vi "Manual Assembly_2.vi"() -> ()   [LabVIEW 2016]
uses:
  Classes/Routine/Routine Enum.ctl
  Classes/Routine/Settings.ctl
  Classes/Assembly/Assembly Run.lvclass
  Classes/Workspace/Fixture Enum.ctl
  Classes/Controller/Controller.lvclass
  Classes/Workspace/Fixture.lvclass
  Classes/Routine/Routine.lvclass
panel:
  in  "Routine type":T1(ring)
  in  "inistialize BT":bool
  out "inistialize":bool
  in  "Routine n":T2(ring)
  in  "Settings":T3
  in  "?":bool
  in  "Update":bool
  in  "Stage":i32(listbox)=-1
  in  "Routine":T4=enum."Dispense on Plate"
  in  "Stop":bool
  in  "Remove":bool
  in  "Add":bool
  in  "Go":bool
  # "6 Inch"
  # "8 Inch"
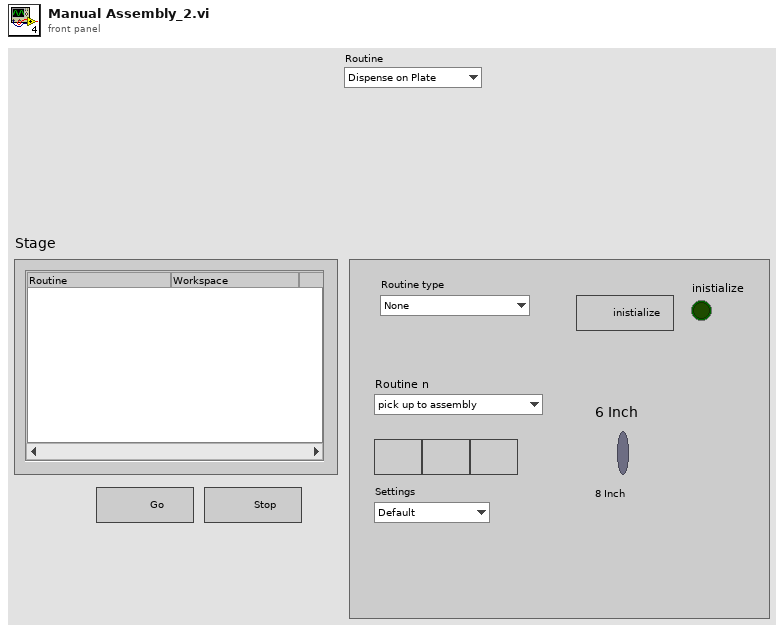
[diagram p1: front panel]
types:
  T1 = enum16{"None", "Kapton assembly", "sensor assembly", "PCB assembly2", "PCB assembly", "Pick up and Put down", "baseplate dispense", "sensor dispense", "sensor dispense2"}
  T2 = enum16{"pick up to assembly", "put down pick up tool", "Primary Pick Up", "Pick Up All", "Put Down Secondary", "Put Down All", "Release Syringe", "Secondary Pick Up", "Secure Syringe", "Dispense on Plate", "Dispense on Kapton", "Dispense on Sensor", "Dispense on Sensor2"}
  T3 = typedef "Routine.lvclass/Settings.ctl" = enum16{"Default", "Custom"}
  T4 = typedef "Routine.lvclass/Routine Enum.ctl" = enum16{"Primary Pick Up", "Pick Up All", "Put Down Secondary", "Put Down All", "Release Syringe", "Secondary Pick Up", "Secure Syringe", "Dispense on Plate", "Dispense on Kapton", "Dispense on Sensor", "Dispense on Sensor2"}
  T5 = typedef "Fixture.lvclass/Fixture Enum.ctl" = enum16{"Assembly Tray", "Syringe Space", "Component", "Pick Up Tool", "Current Position"}
  T6 = enum16{"pick up to assembly", "put down pick up tool", "Primary Pick Up", "Pick Up All", "Put Down Secondary", "Put Down All", "Release Syringe", "Secondary Pick Up", "Secure Syringe", "Dispense on Plate", "Dispense on Kapton", "Dispense on Sensor", "Dispense on Sensor2"}[]
  T7 = typedef "Controller.lvclass/Controllers.ctl" = cluster{"I-O.lvclass":refnum<class "I-O.lvclass">, "Motion.lvclass":refnum<class "Motion.lvclass">, "Dispenser.lvclass":refnum<class "Dispenser.lvclass">}
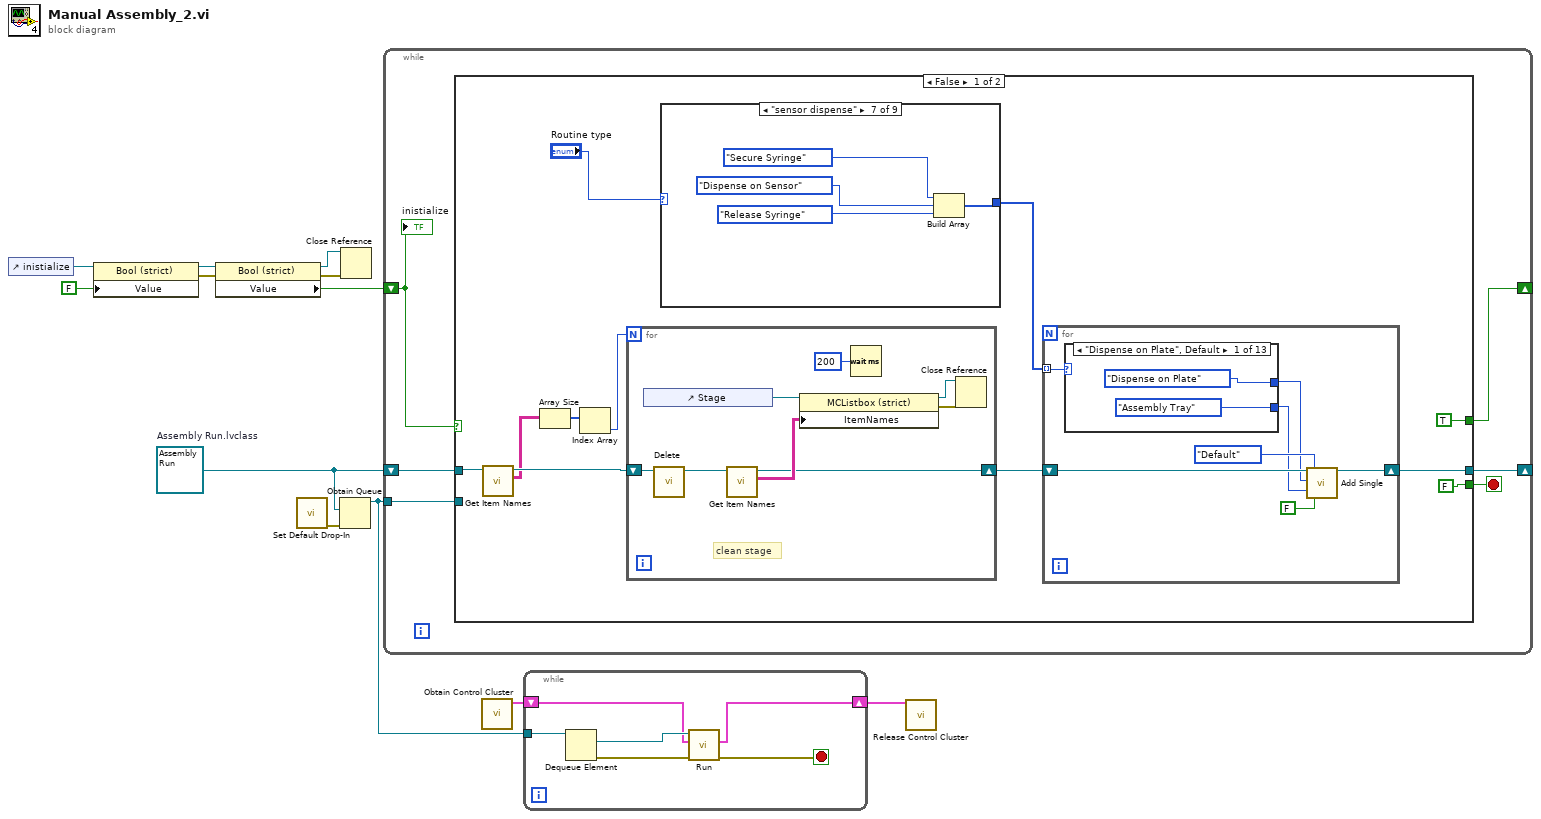
[diagram p0: block diagram]
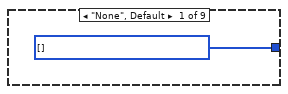
[diagram p2: hidden frame]
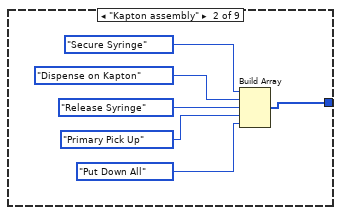
[diagram p3: hidden frame]
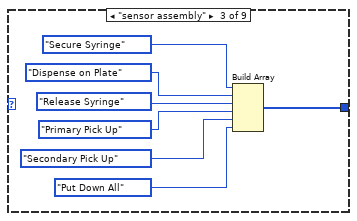
[diagram p4: hidden frame]
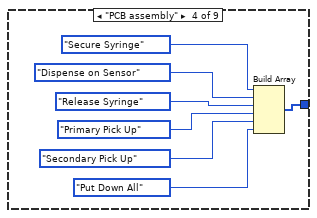
[diagram p5: hidden frame]
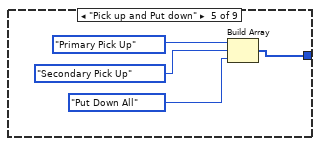
[diagram p6: hidden frame]
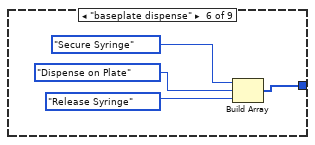
[diagram p7: hidden frame]
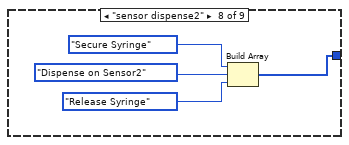
[diagram p8: hidden frame]
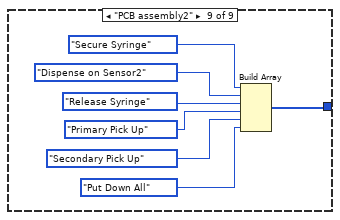
[diagram p9: hidden frame]
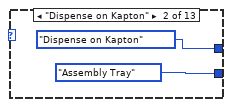
[diagram p10: hidden frame]
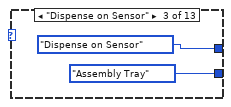
[diagram p11: hidden frame]
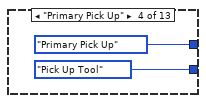
[diagram p12: hidden frame]
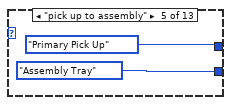
[diagram p13: hidden frame]
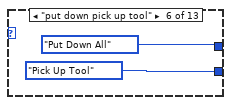
[diagram p14: hidden frame]
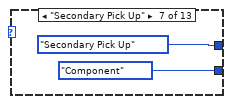
[diagram p15: hidden frame]
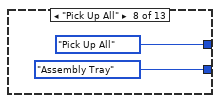
[diagram p16: hidden frame]
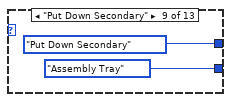
[diagram p17: hidden frame]
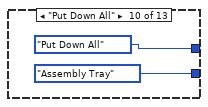
[diagram p18: hidden frame]
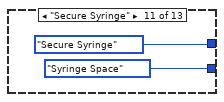
[diagram p19: hidden frame]
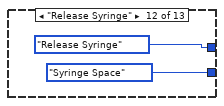
[diagram p20: hidden frame]
diagram:
  w8 = refnum<class "Assembly Run.lvclass"> refnum  # Assembly Run.lvclass
  n1 = control-ref of="inistialize"() -> (w2:refnum<vi>)
  n2 = property class="Bool (strict)"(reference=w2, "Value"=FALSE) -> (reference out=w4:refnum<vi>, error out=w3:errorcluster)  [unwired: 1 in]
  n3 = property class="Bool (strict)"(reference=w4, error in=w3) -> (reference out=w5:refnum<vi>, error out=w6:errorcluster, "Value"=w7:bool)
  n4 = call "Set Default Drop-In.vi"() -> ("error out"=w9:errorcluster)  [unwired: 11 in]
  n5 = Obtain Queue(element data type=w8, error in (no error)=w9) -> (queue out=w12:refnum<queue>)  [unwired: 3 in, 2 out]
  n6 = Close Reference(reference=w5, error in (no error)=w6) -> ()  [unwired: 1 out]
  n7 = while {
    shift-right: [w15] -> _
    shift-left: w8 -> [w16]
    tunnel: w12 -> [w17]
    shift-right: [w13] -> _
    shift-left: w7 -> [w14]
    stop <- w18 stop-if-true
    n8 = case shown="False" w14 {
      selector: w14 -> [_ w117]
      tunnel: [FALSE w125] -> w18
      tunnel: w17 -> [_ w124]
      tunnel: w16 -> [w26 w121]
      tunnel: [w21 w119] -> w15
      tunnel: [TRUE w118] -> w13
      frame False {
        n9 = call "Get Item Names.vi"("Assembly Run in"=w26) -> ("Item names"=w25:string[][], "Assembly Run out"=w27:refnum<class "Assembly Run.lvclass">)  [unwired: 8 in, 1 out]
        n10 = Array Size(array=w25) -> (size(s)=w24:i32[])
        n11 = Index Array(array=w24) -> (element=w23:i32)  [unwired: 1 in]
        n12 = for {
          N: w23 -> [_]
          shift-right: [w108] -> w22
          shift-left: w27 -> [w110]
          # "clean stage"
          n13 = control-ref of="Stage"() -> (w107:refnum<vi>)
          n14 = call "Delete.vi"("Assembly In"=w110) -> ("Assembly Out"=w109:refnum<class "Assembly Run.lvclass">)  [unwired: 9 in, 1 out]
          n15 = call "Get Item Names.vi"("Assembly Run in"=w109) -> ("Item names"=w113:string[][], "Assembly Run out"=w108:refnum<class "Assembly Run.lvclass">)  [unwired: 8 in, 1 out]
          n16 = property class="MCListbox (strict)"(reference=w107, "ItemNames"=w113) -> (reference out=w114:refnum<vi>, error out=w112:errorcluster)  [unwired: 1 in]
          n17 = Wait (ms)(milliseconds to wait=u32 200) -> ()  [unwired: 1 out]
          n18 = Close Reference(reference=w114, error in (no error)=w112) -> ()  [unwired: 1 out]
        }
        n19 = case shown="\"sensor dispense\"" "Routine type" {
          tunnel: [w30 w36 w43 w50 w54 w58 w62 w66 w73] -> w19
          frame "None", Default {
            w30 = T6 [] items=["pick up to assembly", "put down pick up tool", "Primary Pick Up", "Pick Up All", "Put Down Secondary", "Put Down All", "Release Syringe", "Secondary Pick Up", "Secure Syringe", "Dispense on Plate", "Dispense on Kapton", "Dispense on Sensor", "Dispense on Sensor2"]
          }
          frame "Kapton assembly" {
            n20 = Build Array(T2."Secure Syringe" ("Routine n"), T2."Dispense on Kapton" ("Routine n"), T2."Release Syringe" ("Routine n"), T2."Primary Pick Up" ("Routine n"), T2."Put Down All" ("Routine n")) -> (w36:T6)
          }
          frame "sensor assembly" {
            n21 = Build Array(T2."Secure Syringe" ("Routine n"), T2."Dispense on Plate" ("Routine n"), T2."Release Syringe" ("Routine n"), T2."Primary Pick Up" ("Routine n"), T2."Secondary Pick Up" ("Routine n"), T2."Put Down All" ("Routine n")) -> (w43:T6)
          }
          frame "PCB assembly" {
            n22 = Build Array(T2."Secure Syringe" ("Routine n"), T2."Dispense on Sensor" ("Routine n"), T2."Release Syringe" ("Routine n"), T2."Primary Pick Up" ("Routine n"), T2."Secondary Pick Up" ("Routine n"), T2."Put Down All" ("Routine n")) -> (w50:T6)
          }
          frame "Pick up and Put down" {
            n23 = Build Array(T2."Primary Pick Up" ("Routine n"), T2."Secondary Pick Up" ("Routine n"), T2."Put Down All" ("Routine n")) -> (w54:T6)
          }
          frame "baseplate dispense" {
            n24 = Build Array(T2."Secure Syringe" ("Routine n"), T2."Dispense on Plate" ("Routine n"), T2."Release Syringe" ("Routine n")) -> (w58:T6)
          }
          frame "sensor dispense" {
            n25 = Build Array(T2."Secure Syringe" ("Routine n"), T2."Dispense on Sensor" ("Routine n"), T2."Release Syringe" ("Routine n")) -> (w62:T6)
          }
          frame "sensor dispense2" {
            n26 = Build Array(T2."Secure Syringe" ("Routine n"), T2."Dispense on Sensor2" ("Routine n"), T2."Release Syringe" ("Routine n")) -> (w66:T6)
          }
          frame "PCB assembly2" {
            n27 = Build Array(T2."Secure Syringe" ("Routine n"), T2."Dispense on Sensor2" ("Routine n"), T2."Release Syringe" ("Routine n"), T2."Primary Pick Up" ("Routine n"), T2."Secondary Pick Up" ("Routine n"), T2."Put Down All" ("Routine n")) -> (w73:T6)
          }
        }
        n28 = for {
          shift-right: [w80] -> w21
          shift-left: w22 -> [w79]
          tunnel: w19 -> [w76] mode=indexing
          n29 = case shown="\"Dispense on Plate\", Default" w76 {
            tunnel: [Fixture_Enum."Assembly Tray" ("Fixture") Fixture_Enum."Assembly Tray" ("Fixture") Fixture_Enum."Assembly Tray" ("Fixture") Fixture_Enum."Pick Up Tool" ("Fixture") Fixture_Enum."Assembly Tray" ("Fixture") Fixture_Enum."Pick Up Tool" ("Fixture") Fixture_Enum."Component" ("Fixture") Fixture_Enum."Assembly Tray" ("Fixture") Fixture_Enum."Assembly Tray" ("Fixture") Fixture_Enum."Assembly Tray" ("Fixture") Fixture_Enum."Syringe Space" ("Fixture") Fixture_Enum."Syringe Space" ("Fixture") Fixture_Enum."Assembly Tray" ("Fixture")] -> w75
            tunnel: [Routine_Enum."Dispense on Plate" ("Routine") Routine_Enum."Dispense on Kapton" ("Routine") Routine_Enum."Dispense on Sensor" ("Routine") Routine_Enum."Primary Pick Up" ("Routine") Routine_Enum."Primary Pick Up" ("Routine") Routine_Enum."Put Down All" ("Routine") Routine_Enum."Secondary Pick Up" ("Routine") Routine_Enum."Pick Up All" ("Routine") Routine_Enum."Put Down Secondary" ("Routine") Routine_Enum."Put Down All" ("Routine") Routine_Enum."Secure Syringe" ("Routine") Routine_Enum."Release Syringe" ("Routine") Routine_Enum."Dispense on Sensor2" ("Routine")] -> w74
            frame "Dispense on Plate", Default {
            }
            frame "Dispense on Kapton" {
            }
            frame "Dispense on Sensor" {
            }
            frame "Primary Pick Up" {
            }
            frame "pick up to assembly" {
            }
            frame "put down pick up tool" {
            }
            frame "Secondary Pick Up" {
            }
            frame "Pick Up All" {
            }
            frame "Put Down Secondary" {
            }
            frame "Put Down All" {
            }
            frame "Secure Syringe" {
            }
            frame "Release Syringe" {
            }
            frame "Dispense on Sensor2" {
            }
          }
          n30 = call-dynamic "Add Single.vi"("UI in"=w79, "Routine"=w74, "Fixture"=w75, "Settings"=Settings."Default", "Module Size"=FALSE) -> ("UI out"=w80:refnum<class "Assembly Run.lvclass">)  [unwired: 13 in, 1 out]
        }
      }
      frame True {
        n31 = call "Get Item Names.vi"("Assembly Run in"=w121) -> ("Item names"=w123:string[][], "Assembly Run out"=w120:refnum<class "Assembly Run.lvclass">)  [unwired: 8 in, 1 out]
        n32 = control-ref of="Stage"() -> (w122:refnum<vi>)
        n33 = property class="MCListbox (strict)"(reference=w122, "ItemNames"=w123) -> (reference out=w116:refnum<vi>, error out=w115:errorcluster)  [unwired: 1 in]
        n34 = event shown="[3] \"Add\": Value Change" {
          selector: _ -> [_ _ _ _ _ _]
          dyn-events: _ -> [_ _ _ _ _ _]
          timeout: _ -> [_ _ _ _ _ _]
          tunnel: [_ TRUE _ _ _ _] -> w125
          tunnel: w120 -> [w128 w132 w138 w146 w176 w178]
          tunnel: [w127 w132 w137 w145 w175 w178] -> w119
          tunnel: w124 -> [w129 w131 _ _ _ _]
          tunnel: [w126 w130 w134 w139 w173 FALSE ("inistialize BT")] -> w118
          tunnel: w117 -> [w126 w130 w134 w139 w173 _]
          event "Go": Value Change {
            w127 = refnum<class "Assembly Run.lvclass"> refnum  # Assembly Run.lvclass
            n35 = event-data() -> ()  [unwired: 1 in, 6 out]
            n36 = Enqueue Element(queue=w129, element=w128) -> ()  [unwired: 2 in, 3 out]
          }
          event "Stop": Value Change {
            n37 = event-data() -> ()  [unwired: 1 in, 6 out]
            n38 = Release Queue(queue=w131) -> ()  [unwired: 2 in, 3 out]
          }
          event "Update": Value Change {
            n39 = event-data() -> ()  [unwired: 1 in, 6 out]
            n40 = local read "Routine"() -> (w136:T4)
            n41 = local read "Stage"() -> (w135:i32)
            n42 = call "Update.vi"("Row"=w135, "Routine"=w136, "Assembly Run in"=w138) -> ("Assembly Run out"=w137:refnum<class "Assembly Run.lvclass">)  [unwired: 7 in, 1 out]
          }
          event "Add": Value Change {
            n43 = event-data() -> ()  [unwired: 1 in, 1 out]
            n44 = case shown="\"Dispense on Sensor2\"" "Routine n" {
              tunnel: [Fixture_Enum."Assembly Tray" ("Fixture") Fixture_Enum."Assembly Tray" ("Fixture") Fixture_Enum."Assembly Tray" ("Fixture") Fixture_Enum."Pick Up Tool" ("Fixture") Fixture_Enum."Assembly Tray" ("Fixture") Fixture_Enum."Pick Up Tool" ("Fixture") Fixture_Enum."Component" ("Fixture") Fixture_Enum."Assembly Tray" ("Fixture") Fixture_Enum."Assembly Tray" ("Fixture") Fixture_Enum."Assembly Tray" ("Fixture") Fixture_Enum."Syringe Space" ("Fixture") Fixture_Enum."Syringe Space" ("Fixture") Fixture_Enum."Assembly Tray" ("Fixture")] -> w143
              tunnel: [Routine_Enum."Dispense on Plate" ("Routine") Routine_Enum."Dispense on Kapton" ("Routine") Routine_Enum."Dispense on Sensor" ("Routine") Routine_Enum."Primary Pick Up" ("Routine") Routine_Enum."Primary Pick Up" ("Routine") Routine_Enum."Put Down All" ("Routine") Routine_Enum."Secondary Pick Up" ("Routine") Routine_Enum."Pick Up All" ("Routine") Routine_Enum."Put Down Secondary" ("Routine") Routine_Enum."Put Down All" ("Routine") Routine_Enum."Secure Syringe" ("Routine") Routine_Enum."Release Syringe" ("Routine") Routine_Enum."Dispense on Sensor2" ("Routine")] -> w140
              frame "Dispense on Plate", Default {
              }
              frame "Dispense on Kapton" {
              }
              frame "Dispense on Sensor" {
              }
              frame "Primary Pick Up" {
              }
              frame "pick up to assembly" {
              }
              frame "put down pick up tool" {
              }
              frame "Secondary Pick Up" {
              }
              frame "Pick Up All" {
              }
              frame "Put Down Secondary" {
              }
              frame "Put Down All" {
              }
              frame "Secure Syringe" {
              }
              frame "Release Syringe" {
              }
              frame "Dispense on Sensor2" {
              }
            }
            n45 = call-dynamic "Add Single.vi"("UI in"=w146, "Routine"=w140, "Fixture"=w143, "Settings"="Settings", "Module Size"="?") -> ("UI out"=w145:refnum<class "Assembly Run.lvclass">)  [unwired: 13 in, 1 out]
          }
          event "Remove": Value Change {
            n46 = event-data() -> ()  [unwired: 1 in, 6 out]
            n47 = call "Delete.vi"("Index"="Stage", "Assembly In"=w176) -> ("Assembly Out"=w175:refnum<class "Assembly Run.lvclass">)  [unwired: 8 in, 1 out]
          }
          event "inistialize BT": Value Change {
            n48 = event-data() -> ()  [unwired: 1 in, 6 out]
          }
        }
        n49 = Close Reference(reference=w116, error in (no error)=w115) -> ()  [unwired: 1 out]
      }
    }
    "inistialize" <- w14
  }
  n50 = call "Obtain Control Cluster.vi"() -> ("Control Out"=w11:T7)  [unwired: 11 in]
  n51 = while {
    tunnel: w12 -> [w184]
    shift-right: [w179] -> w10
    shift-left: w11 -> [w182]
    stop <- w180 stop-if-true
    n52 = Dequeue Element(queue=w184) -> (element=w183:refnum<class "Assembly Run.lvclass">, error out=w181:errorcluster)  [unwired: 2 in, 2 out]
    n53 = call-dynamic "Run.vi"("error in (no error)"=w181, "Control In"=w182, "Assembly In"=w183) -> ("error out"=w180:errorcluster, "Control Out"=w179:T7)  [unwired: 6 in, 1 out]
  }
  n54 = call "Release Control Cluster.vi"("output cluster"=w10) -> ()  [unwired: 11 in]
